vi "ARDUINO_PRACTICA.vi"() -> ()   [LabVIEW 2021]
uses:
  <vilib>/Instr/_visa.llb/VISA Configure Serial Port (Instr).vi
panel:
  in  "Stop":bool
  out "Serial Buffer":string
  in  "Puerto COM":refnum<visa-resource-name>
  out "Gasolina":dbl(slide) scale=0.0..100.0
  out "Temperatura":dbl(slide) scale=0.0..50.0
  out "Velocidad":dbl(knob) scale=0.0..20.0
  out "Bateria":dbl(knob) scale=0.0..10.0
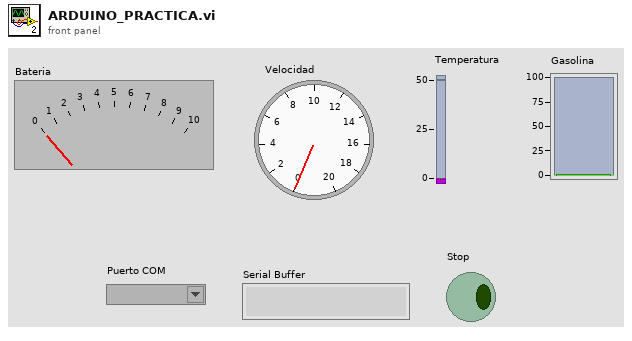
[diagram p1: front panel]
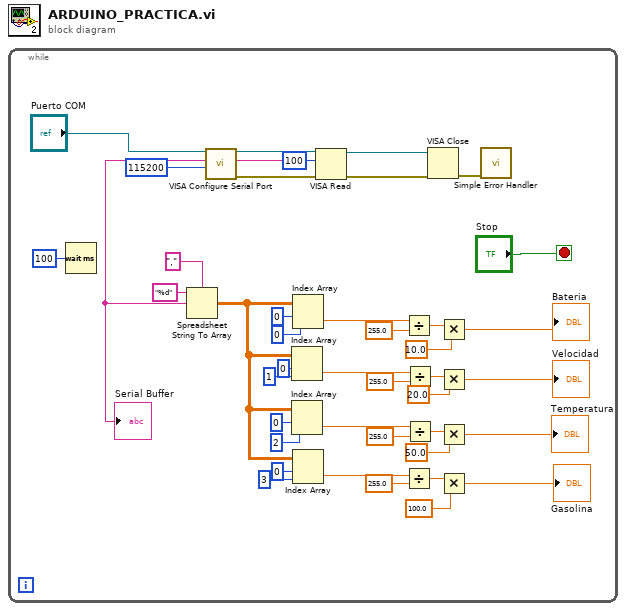
[diagram p0: block diagram]
diagram:
  n1 = while {
    stop <- "Stop" stop-if-true
    n2 = Wait (ms)(milliseconds to wait=u32 100) -> ()  [unwired: 1 out]
    n3 = call-poly "VISA Configure Serial Port"("VISA resource name"="Puerto COM", "baud rate (9600)"=u32 115200) -> ("VISA resource name out"=w40:refnum<visa-resource-name>, "error out"=w39:errorcluster)  [unwired: 12 in]
    n4 = VISA Read(VISA resource name=w40, byte count=u32 100, error in (no error)=w39) -> (VISA resource name out=w37:refnum<visa-resource-name>, read buffer=w32:string, error out=w36:errorcluster)  [unwired: 1 out]
    "Serial Buffer" <- w32
    n5 = Spreadsheet String To Array(delimiter (Tab)=",", format string="%d", spreadsheet string=w32) -> (array=w29:dbl[][])  [unwired: 1 in]
    n6 = Index Array(array=w29, index (row)=0 ("disabled index (row)"), index (col)=1 ("disabled index (col)")) -> (element=w19:dbl)
    n7 = Index Array(array=w29, index (row)=0, index (col)=2 ("disabled index (col)")) -> (element=w18:dbl)
    n8 = Index Array(array=w29, index (row)=0, index (col)=0 ("disabled index (col)")) -> (element=w20:dbl)
    n9 = Index Array(array=w29, index (row)=0, index (col)=3 ("disabled index (col)")) -> (element=w17:dbl)
    n10 = Divide(x=w20, y=255.0) -> (x/y=w12:dbl)
    n11 = Divide(x=w17, y=255.0) -> (x/y=w9:dbl)
    n12 = Divide(x=w19, y=255.0) -> (x/y=w11:dbl)
    n13 = Divide(x=w18, y=255.0) -> (x/y=w10:dbl)
    n14 = VISA Close(VISA resource name=w37, error in (no error)=w36) -> (error out=w34:errorcluster)
    n15 = Multiply(x=w12, y=10.0) -> (x*y=→"Bateria":dbl)
    n16 = Multiply(x=w11, y=20.0) -> (x*y=→"Velocidad":dbl)
    n17 = Multiply(x=w10, y=50.0) -> (x*y=→"Temperatura":dbl)
    n18 = Multiply(x=w9, y=100.0) -> (x*y=→"Gasolina":dbl)
    n19 = call <vilib>:"Simple Error Handler.vi"("error in (no error)"=w34) -> ()  [unwired: 4 in, 5 out]
  }
